vi "FTW-Subscription-Worker.vi"(0 "Backend Handler":refnum<user-event>, 2 "SUB Socket":refnum<class "FTW-Socket.lvclass">) -> ()   [LabVIEW 2014, in "FTW-Subscription.lvclass"]
uses:
  FTW-Subscription.lvclass
  socket/FTW-Socket.lvclass
panel:
  out "recv err":errorcluster
  out "Iteration":i32
  out "Incoming Messages":i32
  # "Inputs"
  # "Debug"
  # "Outputs"
  # "This asynchronous worker has no outputs"
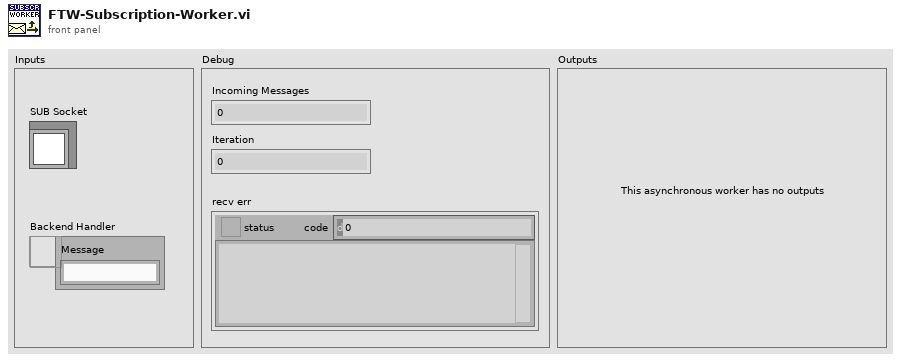
[diagram p1: front panel]
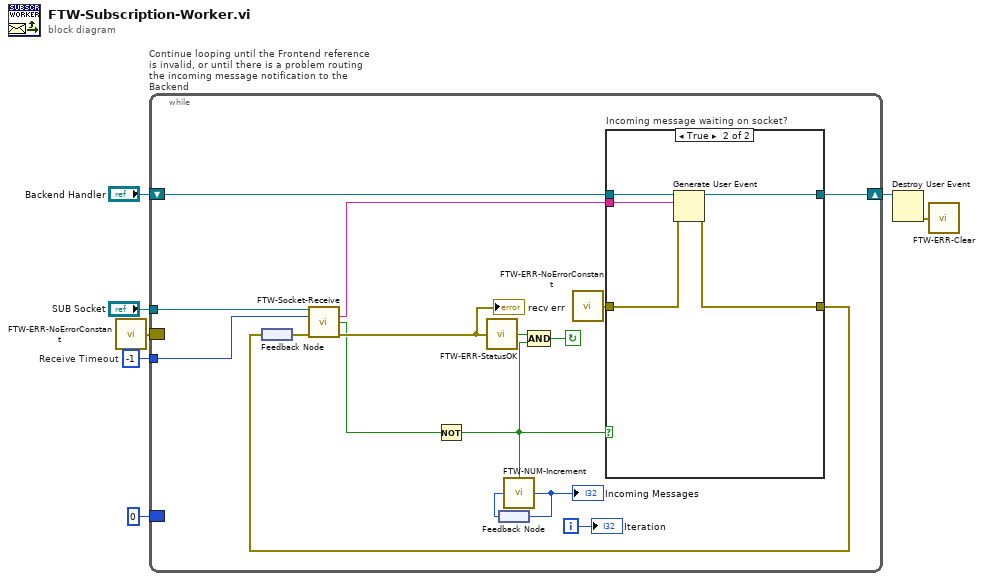
[diagram p0: block diagram]
diagram:
  w2 = -1  # Receive Timeout
  n1 = call "FTW-ERR-NoErrorConstant.vi"() -> ("no error"=w1:errorcluster)
  n2 = while "Continue looping until the Frontend reference is invalid, or until there is a problem routing the incoming message notification to the Backend" {
    border: w1 -> [_]
    shift-right: [w21] -> w6
    shift-left: "Backend Handler" -> [w23]
    border: 0 ("Messages Handled") -> [_]
    tunnel: "SUB Socket" -> [w13]
    tunnel: w2 -> [w8]
    i -> [w19]
    stop <- w15 continue-if-true
    n3 = feedback #1() -> (w10:errorcluster)
    n4 = call "FTW-Socket-Receive.vi"("FTW Socket"=w13, "Timeout"=w8, "error in"=w10) -> ("Message"=w11:string, "Timed out?"=w9:bool, "error out"=w12:errorcluster)  [unwired: 9 in, 1 out]
    "recv err" <- w12
    n5 = Not(x=w9) -> (.not. x?=w14:bool)
    n6 = call "FTW-ERR-StatusOK.vi"("error to check"=w12) -> ("Status OK?"=w16:bool)
    n7 = feedback #2() -> (w17:i32)
    n8 = call "FTW-NUM-Increment.vi"("Initial Value"=w17, "Increment?"=w14) -> ("Final Value"=w18:i32)
    "Incoming Messages" <- w18
    n9 = feedback-in #2(w18) -> ()
    n10 = Compound Arithmetic op=AND(w16, w14) -> (w15:bool)
    n11 = call "FTW-ERR-NoErrorConstant.vi"() -> ("no error"=w20:errorcluster)
    n12 = case "Incoming message waiting on socket?" shown="True" w14 {
      tunnel: w23 -> [w25 w30]
      tunnel: [w24 w28] -> w22
      tunnel: [w25 w29] -> w21
      tunnel: w20 -> [w24 w27]
      tunnel: w11 -> [_ w26]
      frame False {
      }
      frame True {
        n13 = Generate User Event(user event=w30, event data cluster=w26, error in=w27) -> (user event out=w29:refnum<user-event>, error out=w28:errorcluster)  [unwired: 1 in]
      }
    }
    n14 = feedback-in #1(w22) -> ()
    "Iteration" <- w19
  }
  n15 = Destroy User Event(user event=w6) -> (error out=w4:errorcluster)  [unwired: 1 in]
  n16 = call "FTW-ERR-Clear.vi"("error to snuff"=w4) -> ()  [unwired: 1 out]
